vi "check_result.vi"(9 "RMS":dbl[][](array[numeric]), 10 "measured_value":dbl[][](array[numeric]), 11 "tolerance_list":T1) -> (3 "Array":bool[][](array[boolean]))   [LabVIEW 2017]
uses:
  types/tolerance_list.ctl
  types/tolerance.ctl
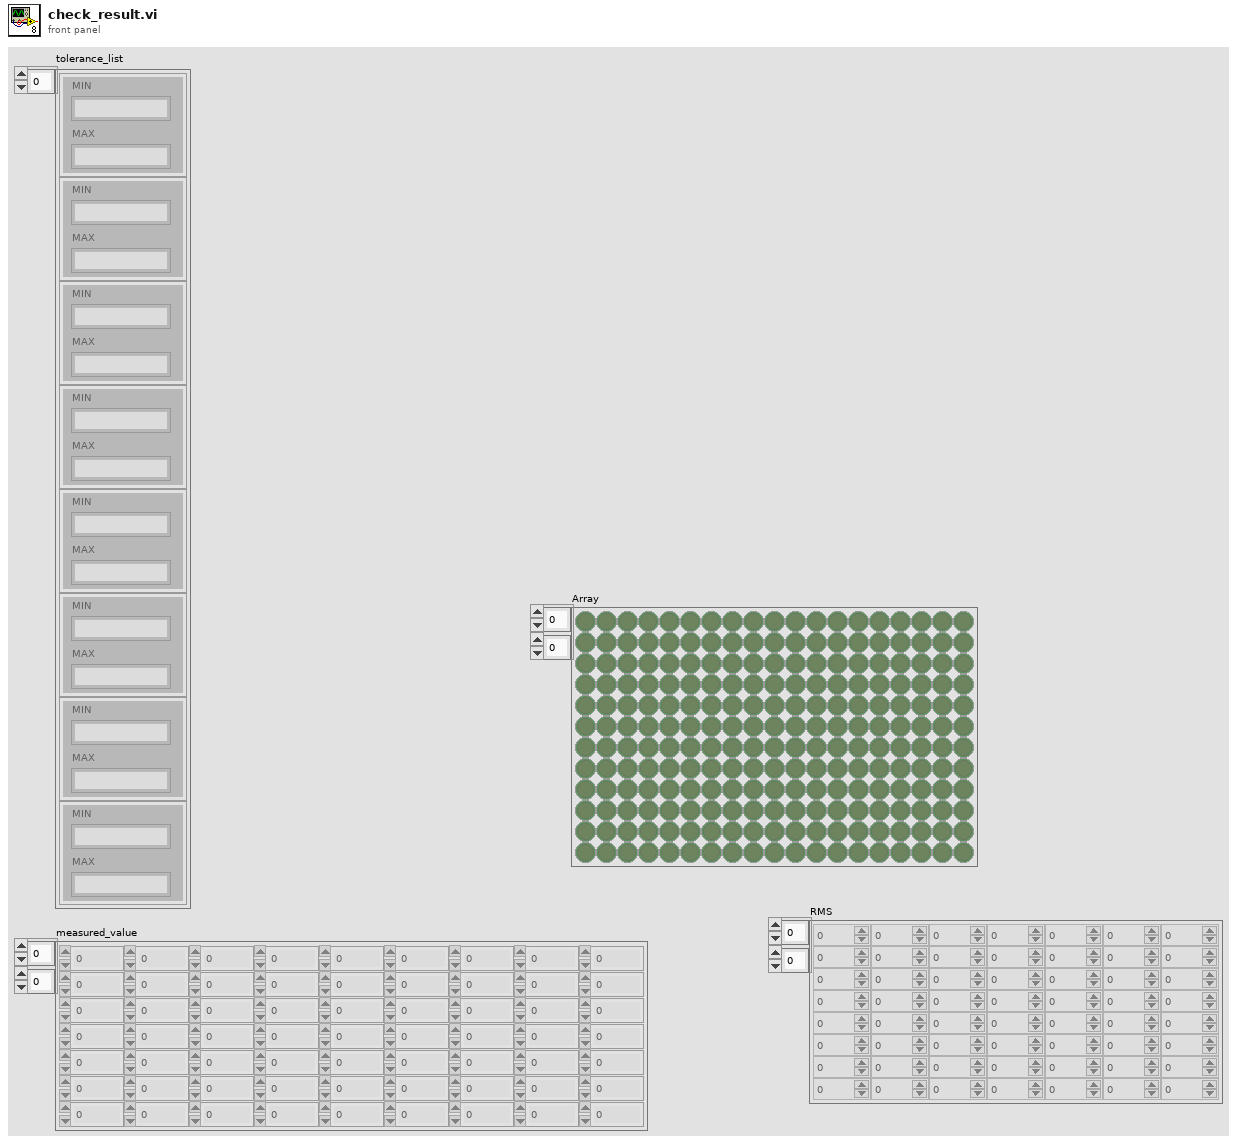
[diagram p1: front panel]
types:
  T1 = typedef "tolerance_list.ctl" = T2[]
  T2 = typedef "tolerance.ctl" = cluster{"MIN":string, "MAX":string}
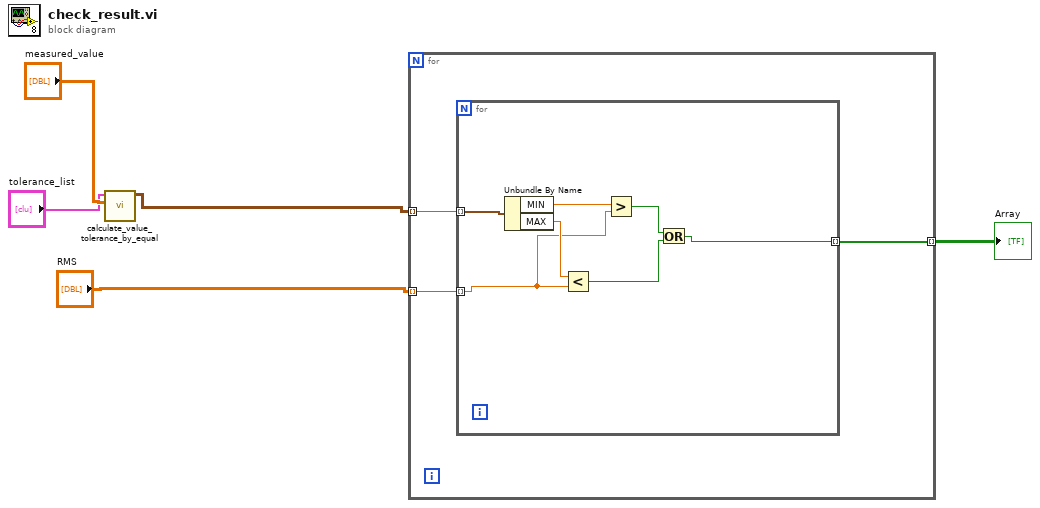
[diagram p0: block diagram]
diagram:
  n1 = call "calculate_value_tolerance_by_equal.vi"("measured_value"="measured_value", "tolerance_list"="tolerance_list") -> ("Array"=w3:cluster{"MIN":dbl, "MAX":dbl}[][])  [unwired: 9 in]
  n2 = for {
    tunnel: w3 -> [w8] mode=indexing
    tunnel: "RMS" -> [w7] mode=indexing
    tunnel: [w6] -> w1 mode=indexing
    n3 = for {
      tunnel: w8 -> [w15] mode=indexing
      tunnel: w7 -> [w12] mode=indexing
      tunnel: [w9] -> w6 mode=indexing
      n4 = Unbundle By Name(w15) -> ("MIN"=w13:dbl, "MAX"=w14:dbl)
      n5 = Less?(x=w14, y=w12) -> (x < y?=w10:bool)
      n6 = Greater?(x=w13, y=w12) -> (0:w11:bool)
      n7 = Or(x=w11, y=w10) -> (x .or. y?=w9:bool)
    }
  }
  "Array" <- w1
